vi "File.CSV Prep, Add Quites to String with Comma.vi"(10 "String In":string) -> (2 "String Out":string)   [LabVIEW 2018]
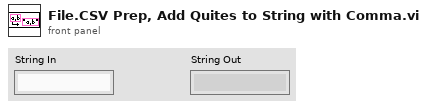
[diagram p1: front panel]
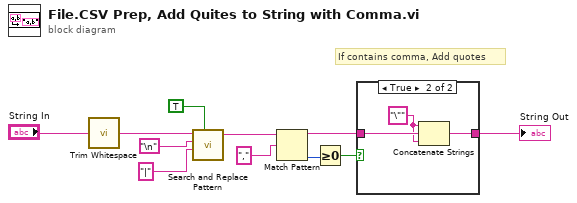
[diagram p0: block diagram]
diagram:
  # "If contains comma, Add quotes"
  n1 = call <vilib>:"Trim Whitespace.vi"("string"="String In") -> ("trimmed string"=w10:string)  [unwired: 1 in]
  n2 = call <vilib>:"Search and Replace Pattern.vi"("string"=w10, "regular expression (\"\")"="\n", "replace string (\"\")"="|", "replace all? (F)"=TRUE) -> ("result string"=w6:string)  [unwired: 1 in, 1 out]
  n3 = Match Pattern(string=w6, regular expression=",") -> (before substring=w2:string, offset past match=w4:i32)  [unwired: 1 in, 2 out]
  n4 = Greater Or Equal To 0?(x=w4) -> (x >= 0?=w3:bool)
  n5 = case shown="True" w3 {
    tunnel: w2 -> [w12 w15]
    tunnel: [w12 w13] -> w1
    frame False {
    }
    frame True {
      w14 = "\""
      n6 = Concatenate Strings(w14, w15, w14) -> (w13:string)
    }
  }
  "String Out" <- w1
